vi "GetSwerveEncoders.vi"() -> (16 "Swerve 0 Velocity (ft/s)":dbl, 17 "Swerve 3 Velocity (ft/s)":dbl, 18 "Swerve 1 Velocity (ft/s)":dbl, 19 "Swerve 2 Velocity (ft/s)":dbl, 20 "Swerve 0 Azimuth Position (deg)":dbl, 22 "Swerve 1 Azimuth Position (deg)":dbl, 24 "Swerve 2 Azimuth Position (deg)":dbl, 26 "Swerve 3 Azimuth Position (deg)":dbl)   [LabVIEW 2020]
doc: "Gets the drive distance, azimuth position, and velocity encoder readings from all of the swerve modules. This VI is also useful for characterizing the drive system allowing for estimation of the robot acceleration and plotting of the module velocities. Deteremines the true shifter state based on photo-interrupter sensors on each module. Please see sensors.vi for a reading of the true robot ground speed (as this must be calculated after using the module odometry VIs)."
uses:
  sensordata.vi
  driverdata.vi
  GRNF_CTREMotor.vi
  <vilib>/Rock Robotics/WPI/ThirdParty/Phoenix-LabVIEW/Motor Controller/Get/CTRE_Phoenix_MotorController_GetSelectedSensorData.vi
  <vilib>/Rock Robotics/WPI/ThirdParty/Phoenix-LabVIEW/Motor Controller/Get/CTRE_Phoenix_MotorController_GetLimitSwitchStates.vi
  <vilib>/Rock Robotics/WPI/ThirdParty/Phoenix-LabVIEW/Motor Controller/Get/CTRE_Phoenix_MotorController_GetGeneralStatus.vi
  GlobalDrivebase.vi
panel:
  in  "Shift Time Threshold (ms)":u32=250
  out "Acceleration (ft/s^2)":dbl format="%.1f"
  in  "Reset Acceleration Test":bool
  in  "Plot and Measure":bool
  out "Drive Encoder Velocities (ft/s)":cluster{dbl, dbl, dbl, dbl}(graph)
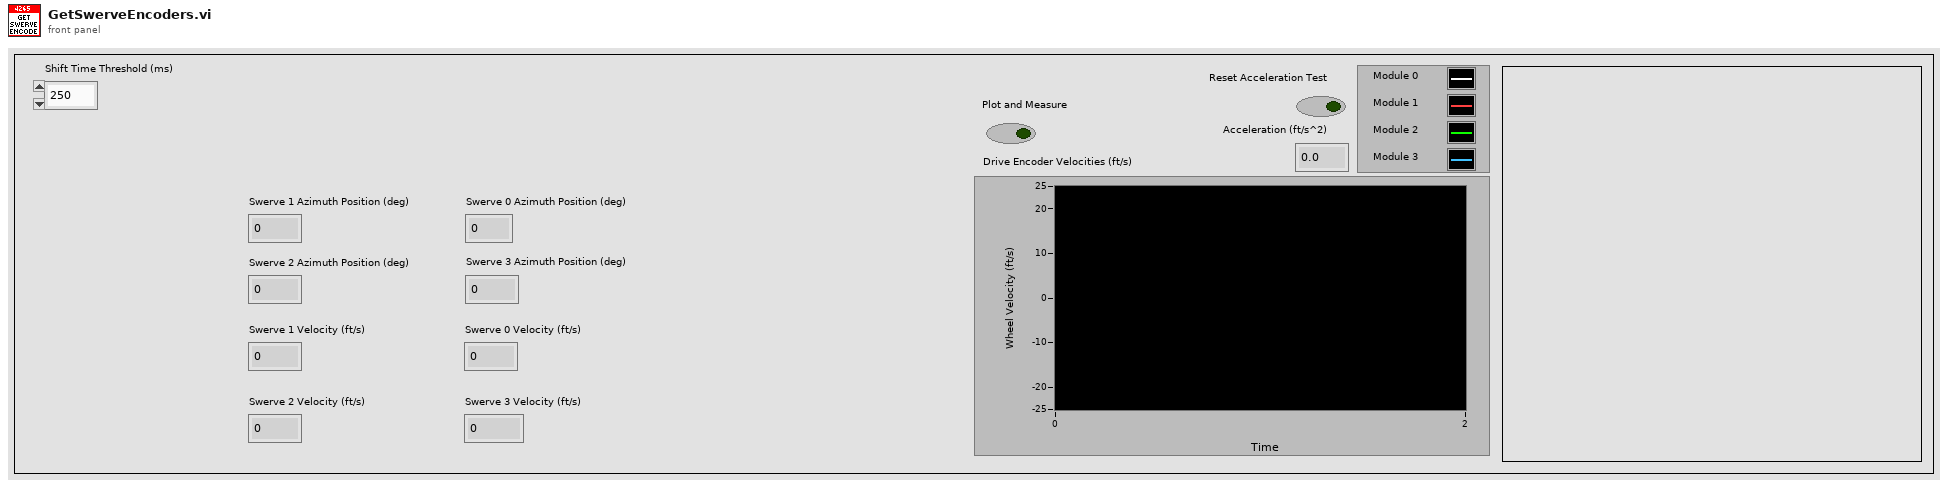
[diagram p1: front panel]
types:
  T1 = typedef "WPI_MotorControlDeviceRef.ctl" = cluster{"DeviceStatus":errorcluster, "Type":T2, "PWM":cluster{"PWM Channel":T3, "DeadBand":T4}, "CAN":cluster{"Device Number":u8, "SetOutput VI Ref":variant, "GetOutput VI Ref":variant, "Enable VI Ref":variant, "Disable VI Ref":variant, "Data":variant}, "Invert":bool, "DIO PWM":cluster{"PWM \"Enable\" Channel":T3, "DIOChannel":T5, "PWM Rate":dbl}}
  T2 = typedef "WPI_MotorControlType.ctl" = enum16{"PWM", "CAN", "DIO PWM"}
  T3 = typedef "FPGA_DIOPWMChannel.ctl" = enum8{"PWM 0", "PWM 1", "PWM 2", "PWM 3", "PWM 4", "PWM 5", "PWM 6", "PWM 7", "PWM 8", "PWM 9", "PWM MXP 0", "PWM MXP 1", "PWM MXP 2", "PWM MXP 3", "PWM MXP 4", "PWM MXP 5", "PWM MXP 6", "PWM MXP 7", "PWM MXP 8", "PWM MXP 9", "Invalid"}
  T4 = typedef "WPI_PWMDeadband.ctl" = cluster{"Name":string, "maxPositivePwm":i32, "minPositivePwm":i32, "centerPwm":i32, "maxNegativePwm":i32, "minNegativePwm":i32, "angularRange":u16}
  T5 = typedef "FPGA_DIOChannel.ctl" = enum8{"DIO 0", "DIO 1", "DIO 2", "DIO 3", "DIO 4", "DIO 5", "DIO 6", "DIO 7", "DIO 8", "DIO 9", "DIO MXP 0", "DIO MXP 1", "DIO MXP 2", "DIO MXP 3", "DIO MXP 4", "DIO MXP 5", "DIO MXP 6", "DIO MXP 7", "DIO MXP 8", "DIO MXP 9", "DIO MXP 10", "DIO MXP 11", "DIO MXP 12", "DIO MXP 13", "DIO MXP 14", "DIO MXP 15", "SPI Port CS1", "SPI Port CS2", "SPI Port CS3", "SPI Port MISO", "SPI Port MOSI", "Invalid"}
  T6 = enum16{"Low Gear", "High Gear", "Transiting", "Unknown", "Force Low Gear"}
  T7 = cluster{"Velocity (ft/s)":dbl, "Velocity (ft/s)":dbl, "Velocity (ft/s)":dbl, "Velocity (ft/s)":dbl}
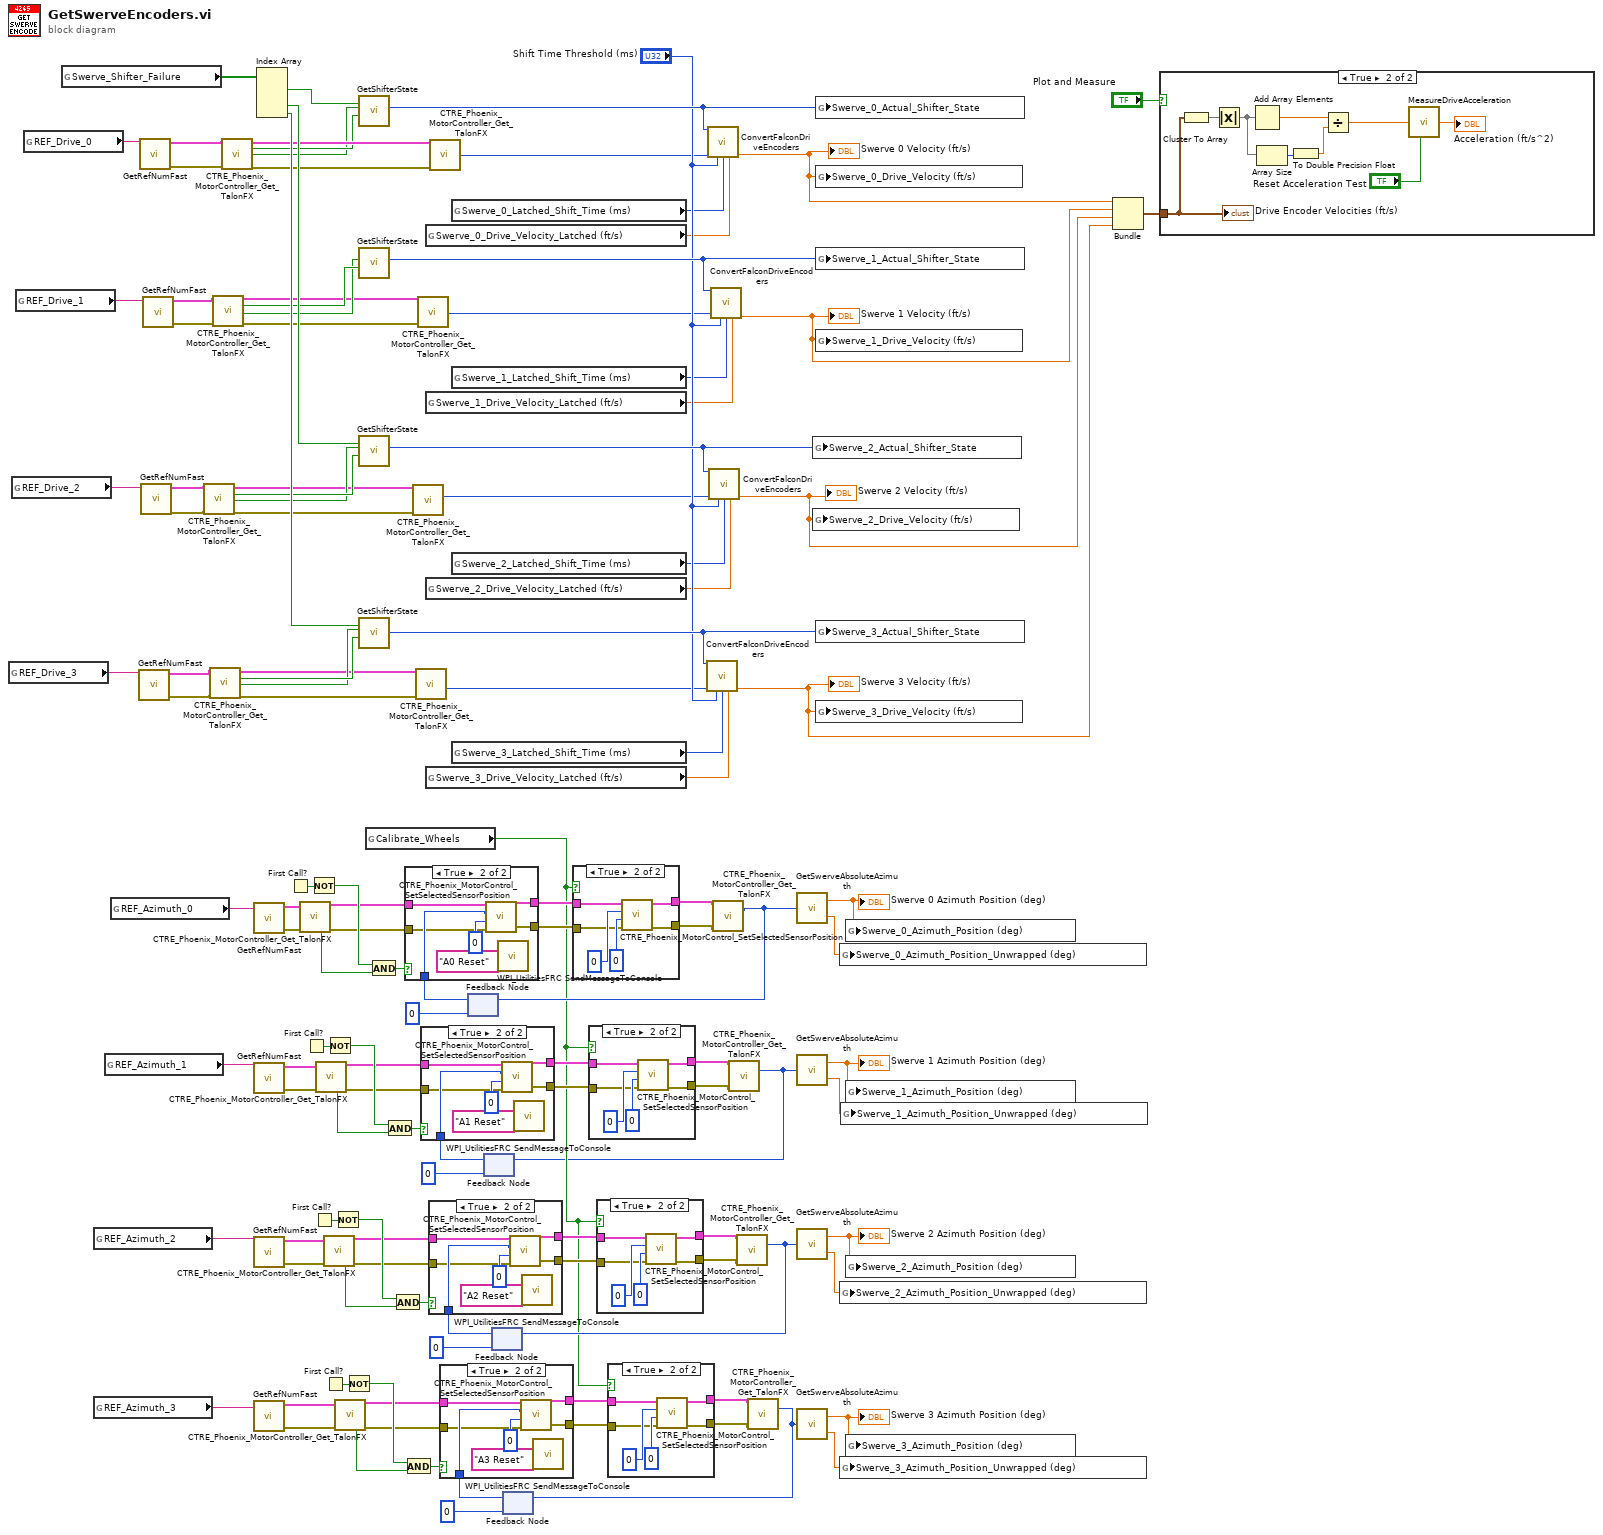
[diagram p0: block diagram]
diagram:
  n1 = global read "GlobalDrivebase.vi" "REF_Drive_3"() -> (w5:string)
  n2 = global read "GlobalDrivebase.vi" "REF_Drive_2"() -> (w6:string)
  n3 = global read "GlobalDrivebase.vi" "REF_Drive_1"() -> (w7:string)
  n4 = global read "GlobalDrivebase.vi" "REF_Drive_0"() -> (w8:string)
  n5 = global read "sensordata.vi" "Swerve_Shifter_Failure"() -> (w122:bool[])
  n6 = global read "GlobalDrivebase.vi" "REF_Azimuth_2"() -> (w2:string)
  n7 = global read "GlobalDrivebase.vi" "REF_Azimuth_3"() -> (w1:string)
  n8 = global read "GlobalDrivebase.vi" "REF_Azimuth_1"() -> (w3:string)
  n9 = global read "GlobalDrivebase.vi" "REF_Azimuth_0"() -> (w4:string)
  n10 = call-poly "GetRefNumFast.vi"("RefNum Name"=w5) -> ("Error"=w16:errorcluster, "Device Reference"=w15:T1)  [unwired: 5 in]
  n11 = call-poly "GetRefNumFast.vi"("RefNum Name"=w8) -> ("Error"=w34:errorcluster, "Device Reference"=w33:T1)  [unwired: 5 in]
  n12 = call-poly "GetRefNumFast.vi"("RefNum Name"=w6) -> ("Error"=w22:errorcluster, "Device Reference"=w21:T1)  [unwired: 5 in]
  n13 = call-poly "GetRefNumFast.vi"("RefNum Name"=w7) -> ("Error"=w31:errorcluster, "Device Reference"=w32:T1)  [unwired: 5 in]
  n14 = call-poly <vilib>:"CTRE_Phoenix_MotorController_Get_TalonFX.vi"("PhoenixMotorControlDevRef"=w21, "error in"=w22) -> ("PhoenixMotorControlDevRef"=w24:T1, "Forward Limit Closed?"=w26:bool, "Reverse Limit Closed?"=w25:bool, "error out"=w23:errorcluster)  [unwired: 10 in]
  n15 = call-poly <vilib>:"CTRE_Phoenix_MotorController_Get_TalonFX.vi"("PhoenixMotorControlDevRef"=w15, "error in"=w16) -> ("PhoenixMotorControlDevRef"=w18:T1, "Forward Limit Closed?"=w20:bool, "Reverse Limit Closed?"=w19:bool, "error out"=w17:errorcluster)  [unwired: 10 in]
  n16 = call-poly <vilib>:"CTRE_Phoenix_MotorController_Get_TalonFX.vi"("PhoenixMotorControlDevRef"=w32, "error in"=w31) -> ("PhoenixMotorControlDevRef"=w28:T1, "Forward Limit Closed?"=w30:bool, "Reverse Limit Closed?"=w29:bool, "error out"=w27:errorcluster)  [unwired: 10 in]
  n17 = call-poly <vilib>:"CTRE_Phoenix_MotorController_Get_TalonFX.vi"("PhoenixMotorControlDevRef"=w33, "error in"=w34) -> ("PhoenixMotorControlDevRef"=w37:T1, "Forward Limit Closed?"=w36:bool, "Reverse Limit Closed?"=w13:bool, "error out"=w35:errorcluster)  [unwired: 10 in]
  n18 = call-poly "GetRefNumFast.vi"("RefNum Name"=w4) -> ("Error"=w93:errorcluster, "Device Reference"=w94:T1)  [unwired: 5 in]
  n19 = call-poly "GetRefNumFast.vi"("RefNum Name"=w3) -> ("Error"=w78:errorcluster, "Device Reference"=w79:T1)  [unwired: 5 in]
  n20 = call-poly "GetRefNumFast.vi"("RefNum Name"=w2) -> ("Error"=w64:errorcluster, "Device Reference"=w65:T1)  [unwired: 5 in]
  n21 = call-poly "GetRefNumFast.vi"("RefNum Name"=w1) -> ("Error"=w49:errorcluster, "Device Reference"=w50:T1)  [unwired: 5 in]
  n22 = Index Array(array=w122) -> (element #1=w121:bool, element #3=w120:bool, element #4=w119:bool)  [unwired: 4 in, 1 out]
  n23 = First Call?() -> (First Call?: T/F=w97:bool)
  n24 = call-poly <vilib>:"CTRE_Phoenix_MotorController_Get_TalonFX.vi"("PhoenixMotorControlDevRef"=w94, "error in"=w93) -> ("PhoenixMotorControlDevRef"=w92:T1, "Has Reset Occurred?"=w90:bool, "error out"=w91:errorcluster)  [unwired: 8 in, 3 out]
  n25 = First Call?() -> (First Call?: T/F=w82:bool)
  n26 = Not(x=w97) -> (.not. x?=w95:bool)
  n27 = First Call?() -> (First Call?: T/F=w68:bool)
  n28 = call-poly <vilib>:"CTRE_Phoenix_MotorController_Get_TalonFX.vi"("PhoenixMotorControlDevRef"=w79, "error in"=w78) -> ("PhoenixMotorControlDevRef"=w77:T1, "Has Reset Occurred?"=w75:bool, "error out"=w76:errorcluster)  [unwired: 8 in, 3 out]
  n29 = First Call?() -> (First Call?: T/F=w53:bool)
  n30 = call-poly <vilib>:"CTRE_Phoenix_MotorController_Get_TalonFX.vi"("PhoenixMotorControlDevRef"=w65, "error in"=w64) -> ("PhoenixMotorControlDevRef"=w63:T1, "Has Reset Occurred?"=w61:bool, "error out"=w62:errorcluster)  [unwired: 8 in, 3 out]
  n31 = Not(x=w82) -> (.not. x?=w80:bool)
  n32 = Not(x=w68) -> (.not. x?=w66:bool)
  n33 = call-poly <vilib>:"CTRE_Phoenix_MotorController_Get_TalonFX.vi"("PhoenixMotorControlDevRef"=w50, "error in"=w49) -> ("PhoenixMotorControlDevRef"=w48:T1, "Has Reset Occurred?"=w46:bool, "error out"=w47:errorcluster)  [unwired: 8 in, 3 out]
  n34 = Not(x=w53) -> (.not. x?=w51:bool)
  n35 = call "GetShifterState.vi"("Sensor Failure"=w121, "Low Gear Sensor"=w36, "High Gear Sensor"=w13) -> ("Actual Shifter State"=w113:T6)  [unwired: 8 in]
  n36 = call "GetShifterState.vi"("Low Gear Sensor"=w30, "High Gear Sensor"=w29) -> ("Actual Shifter State"=w114:T6)  [unwired: 9 in]
  n37 = call "GetShifterState.vi"("Sensor Failure"=w120, "Low Gear Sensor"=w26, "High Gear Sensor"=w25) -> ("Actual Shifter State"=w112:T6)  [unwired: 8 in]
  n38 = call "GetShifterState.vi"("Sensor Failure"=w119, "Low Gear Sensor"=w20, "High Gear Sensor"=w19) -> ("Actual Shifter State"=w111:T6)  [unwired: 8 in]
  n39 = global read "driverdata.vi" "Calibrate_Wheels"() -> (w43:bool)
  n40 = And(x=w95, y=w90) -> (x .and. y?=w98:bool)
  n41 = And(x=w80, y=w75) -> (x .and. y?=w83:bool)
  n42 = And(x=w66, y=w61) -> (x .and. y?=w69:bool)
  n43 = And(x=w51, y=w46) -> (x .and. y?=w54:bool)
  n44 = call-poly <vilib>:"CTRE_Phoenix_MotorController_Get_TalonFX.vi"("PhoenixMotorControlDevRef"=w24, "error in"=w23) -> ("Velocity (Raw Sensor Units per 100 ms)"=w39:i32)  [unwired: 10 in, 3 out]
  n45 = call-poly <vilib>:"CTRE_Phoenix_MotorController_Get_TalonFX.vi"("PhoenixMotorControlDevRef"=w18, "error in"=w17) -> ("Velocity (Raw Sensor Units per 100 ms)"=w38:i32)  [unwired: 10 in, 3 out]
  n46 = call-poly <vilib>:"CTRE_Phoenix_MotorController_Get_TalonFX.vi"("PhoenixMotorControlDevRef"=w28, "error in"=w27) -> ("Velocity (Raw Sensor Units per 100 ms)"=w40:i32)  [unwired: 10 in, 3 out]
  n47 = global read "sensordata.vi" "Swerve_0_Drive_Velocity_Latched (ft/s)"() -> (w108:dbl)
  n48 = global read "sensordata.vi" "Swerve_1_Drive_Velocity_Latched (ft/s)"() -> (w106:dbl)
  n49 = global read "sensordata.vi" "Swerve_2_Drive_Velocity_Latched (ft/s)"() -> (w104:dbl)
  n50 = global read "sensordata.vi" "Swerve_3_Drive_Velocity_Latched (ft/s)"() -> (w102:dbl)
  n51 = call-poly <vilib>:"CTRE_Phoenix_MotorController_Get_TalonFX.vi"("PhoenixMotorControlDevRef"=w37, "error in"=w35) -> ("Velocity (Raw Sensor Units per 100 ms)"=w41:i32)  [unwired: 10 in, 3 out]
  n52 = global read "sensordata.vi" "Swerve_0_Latched_Shift_Time (ms)"() -> (w109:u32)
  n53 = global read "sensordata.vi" "Swerve_1_Latched_Shift_Time (ms)"() -> (w107:u32)
  n54 = global read "sensordata.vi" "Swerve_2_Latched_Shift_Time (ms)"() -> (w105:u32)
  n55 = global read "sensordata.vi" "Swerve_3_Latched_Shift_Time (ms)"() -> (w103:u32)
  n56 = feedback #1(0 ("Position (Raw Sensor Units)")) -> (w101:i32)
  n57 = case shown="True" w98 {
    tunnel: w91 -> [w129 w133]
    tunnel: w92 -> [w130 w136]
    tunnel: [w130 w132] -> w100
    tunnel: [w129 w131] -> w99
    tunnel: w101 -> [_ w135]
    frame False {
    }
    frame True {
      n58 = call <vilib>:"CTRE_Phoenix_MotorControl_SetSelectedSensorPosition.vi"("error in (no error)"=w133, "pidLoopIdx"=u32 0, "New Sensor Position"=w135, "PhoenixMotorControlDevRef"=w136) -> ("error out"=w131:errorcluster, "PhoenixMotorControlDevRef"=w132:T1)  [unwired: 6 in]
      n59 = call <vilib>:"WPI_UtilitiesFRC SendMessageToConsole.vi"("Message"="A0 Reset") -> ()  [unwired: 14 in, 1 out]
    }
  }
  n60 = feedback #2(0 ("Position (Raw Sensor Units)")) -> (w86:i32)
  n61 = case shown="True" w83 {
    tunnel: w76 -> [w138 w142]
    tunnel: w77 -> [w139 w145]
    tunnel: [w139 w141] -> w85
    tunnel: [w138 w140] -> w84
    tunnel: w86 -> [_ w144]
    frame False {
    }
    frame True {
      n62 = call <vilib>:"CTRE_Phoenix_MotorControl_SetSelectedSensorPosition.vi"("error in (no error)"=w142, "pidLoopIdx"=u32 0, "New Sensor Position"=w144, "PhoenixMotorControlDevRef"=w145) -> ("error out"=w140:errorcluster, "PhoenixMotorControlDevRef"=w141:T1)  [unwired: 6 in]
      n63 = call <vilib>:"WPI_UtilitiesFRC SendMessageToConsole.vi"("Message"="A1 Reset") -> ()  [unwired: 14 in, 1 out]
    }
  }
  n64 = feedback #3(0 ("Position (Raw Sensor Units)")) -> (w72:i32)
  n65 = case shown="True" w69 {
    tunnel: w62 -> [w147 w151]
    tunnel: w63 -> [w148 w154]
    tunnel: [w148 w150] -> w71
    tunnel: [w147 w149] -> w70
    tunnel: w72 -> [_ w153]
    frame False {
    }
    frame True {
      n66 = call <vilib>:"CTRE_Phoenix_MotorControl_SetSelectedSensorPosition.vi"("error in (no error)"=w151, "pidLoopIdx"=u32 0, "New Sensor Position"=w153, "PhoenixMotorControlDevRef"=w154) -> ("error out"=w149:errorcluster, "PhoenixMotorControlDevRef"=w150:T1)  [unwired: 6 in]
      n67 = call <vilib>:"WPI_UtilitiesFRC SendMessageToConsole.vi"("Message"="A2 Reset") -> ()  [unwired: 14 in, 1 out]
    }
  }
  n68 = feedback #4(0 ("Position (Raw Sensor Units)")) -> (w57:i32)
  n69 = case shown="True" w54 {
    tunnel: w47 -> [w156 w160]
    tunnel: w48 -> [w157 w163]
    tunnel: [w157 w159] -> w56
    tunnel: [w156 w158] -> w55
    tunnel: w57 -> [_ w162]
    frame False {
    }
    frame True {
      n70 = call <vilib>:"CTRE_Phoenix_MotorControl_SetSelectedSensorPosition.vi"("error in (no error)"=w160, "pidLoopIdx"=u32 0, "New Sensor Position"=w162, "PhoenixMotorControlDevRef"=w163) -> ("error out"=w158:errorcluster, "PhoenixMotorControlDevRef"=w159:T1)  [unwired: 6 in]
      n71 = call <vilib>:"WPI_UtilitiesFRC SendMessageToConsole.vi"("Message"="A3 Reset") -> ()  [unwired: 14 in, 1 out]
    }
  }
  n72 = case shown="True" w43 {
    tunnel: w99 -> [w165 w167]
    tunnel: w100 -> [w166 w170]
    tunnel: [w166 w171] -> w89
    tunnel: [w165 w172] -> w88
    frame False {
    }
    frame True {
      n73 = call <vilib>:"CTRE_Phoenix_MotorControl_SetSelectedSensorPosition.vi"("error in (no error)"=w167, "pidLoopIdx"=u32 0, "New Sensor Position"=0, "PhoenixMotorControlDevRef"=w170) -> ("error out"=w172:errorcluster, "PhoenixMotorControlDevRef"=w171:T1)  [unwired: 6 in]
    }
  }
  n74 = case shown="True" w43 {
    tunnel: w84 -> [w173 w175]
    tunnel: w85 -> [w174 w178]
    tunnel: [w174 w179] -> w74
    tunnel: [w173 w180] -> w73
    frame False {
    }
    frame True {
      n75 = call <vilib>:"CTRE_Phoenix_MotorControl_SetSelectedSensorPosition.vi"("error in (no error)"=w175, "pidLoopIdx"=u32 0, "New Sensor Position"=0, "PhoenixMotorControlDevRef"=w178) -> ("error out"=w180:errorcluster, "PhoenixMotorControlDevRef"=w179:T1)  [unwired: 6 in]
    }
  }
  n76 = case shown="True" w43 {
    tunnel: w70 -> [w181 w183]
    tunnel: w71 -> [w182 w186]
    tunnel: [w182 w187] -> w60
    tunnel: [w181 w188] -> w59
    frame False {
    }
    frame True {
      n77 = call <vilib>:"CTRE_Phoenix_MotorControl_SetSelectedSensorPosition.vi"("error in (no error)"=w183, "pidLoopIdx"=u32 0, "New Sensor Position"=0, "PhoenixMotorControlDevRef"=w186) -> ("error out"=w188:errorcluster, "PhoenixMotorControlDevRef"=w187:T1)  [unwired: 6 in]
    }
  }
  n78 = case shown="True" w43 {
    tunnel: w55 -> [w189 w191]
    tunnel: w56 -> [w190 w194]
    tunnel: [w190 w195] -> w45
    tunnel: [w189 w196] -> w44
    frame False {
    }
    frame True {
      n79 = call <vilib>:"CTRE_Phoenix_MotorControl_SetSelectedSensorPosition.vi"("error in (no error)"=w191, "pidLoopIdx"=u32 0, "New Sensor Position"=0, "PhoenixMotorControlDevRef"=w194) -> ("error out"=w196:errorcluster, "PhoenixMotorControlDevRef"=w195:T1)  [unwired: 6 in]
    }
  }
  n80 = call "ConvertFalconDriveEncoders.vi"("Shifter State"=w111, "Velocity (Raw Sensor Units per 100 ms)"=w38, "Shift Time Threshold (ms)"="Shift Time Threshold (ms)", "Latched Shift Time (ms)"=w103, "Latched Velocity (ft/s)"=w102) -> ("Velocity (ft/s)"=w123:dbl)  [unwired: 10 in]
  "Swerve 3 Velocity (ft/s)" <- w123
  n81 = call "ConvertFalconDriveEncoders.vi"("Shifter State"=w113, "Velocity (Raw Sensor Units per 100 ms)"=w41, "Shift Time Threshold (ms)"="Shift Time Threshold (ms)", "Latched Shift Time (ms)"=w109, "Latched Velocity (ft/s)"=w108) -> ("Velocity (ft/s)"=w127:dbl)  [unwired: 10 in]
  "Swerve 0 Velocity (ft/s)" <- w127
  n82 = call "ConvertFalconDriveEncoders.vi"("Shifter State"=w112, "Velocity (Raw Sensor Units per 100 ms)"=w39, "Shift Time Threshold (ms)"="Shift Time Threshold (ms)", "Latched Shift Time (ms)"=w105, "Latched Velocity (ft/s)"=w104) -> ("Velocity (ft/s)"=w124:dbl)  [unwired: 10 in]
  "Swerve 2 Velocity (ft/s)" <- w124
  n83 = call "ConvertFalconDriveEncoders.vi"("Shifter State"=w114, "Velocity (Raw Sensor Units per 100 ms)"=w40, "Shift Time Threshold (ms)"="Shift Time Threshold (ms)", "Latched Shift Time (ms)"=w107, "Latched Velocity (ft/s)"=w106) -> ("Velocity (ft/s)"=w125:dbl)  [unwired: 10 in]
  "Swerve 1 Velocity (ft/s)" <- w125
  n84 = call-poly <vilib>:"CTRE_Phoenix_MotorController_Get_TalonFX.vi"("PhoenixMotorControlDevRef"=w89, "error in"=w88) -> ("Position (Raw Sensor Units)"=w87:i32)  [unwired: 10 in, 3 out]
  n85 = feedback-in #1(w87) -> ()
  n86 = call-poly <vilib>:"CTRE_Phoenix_MotorController_Get_TalonFX.vi"("PhoenixMotorControlDevRef"=w74, "error in"=w73) -> ("Position (Raw Sensor Units)"=w14:i32)  [unwired: 10 in, 3 out]
  n87 = feedback-in #2(w14) -> ()
  n88 = call-poly <vilib>:"CTRE_Phoenix_MotorController_Get_TalonFX.vi"("PhoenixMotorControlDevRef"=w60, "error in"=w59) -> ("Position (Raw Sensor Units)"=w58:i32)  [unwired: 10 in, 3 out]
  n89 = feedback-in #3(w58) -> ()
  n90 = call-poly <vilib>:"CTRE_Phoenix_MotorController_Get_TalonFX.vi"("PhoenixMotorControlDevRef"=w45, "error in"=w44) -> ("Position (Raw Sensor Units)"=w42:i32)  [unwired: 10 in, 3 out]
  n91 = feedback-in #4(w42) -> ()
  n92 = call "GetSwerveAbsoluteAzimuth.vi"("Relative Position (Raw Sensor Units)"=w87) -> ("Azimuth Position (deg) [-180,+180]"=w115:dbl, "Current Unwrapped Angle (deg) [-Inf,+Inf]"=w12:dbl)
  "Swerve 0 Azimuth Position (deg)" <- w115
  n93 = call "GetSwerveAbsoluteAzimuth.vi"("Relative Position (Raw Sensor Units)"=w14) -> ("Azimuth Position (deg) [-180,+180]"=w116:dbl, "Current Unwrapped Angle (deg) [-Inf,+Inf]"=w11:dbl)
  "Swerve 1 Azimuth Position (deg)" <- w116
  n94 = call "GetSwerveAbsoluteAzimuth.vi"("Relative Position (Raw Sensor Units)"=w58) -> ("Azimuth Position (deg) [-180,+180]"=w117:dbl, "Current Unwrapped Angle (deg) [-Inf,+Inf]"=w10:dbl)
  "Swerve 2 Azimuth Position (deg)" <- w117
  n95 = call "GetSwerveAbsoluteAzimuth.vi"("Relative Position (Raw Sensor Units)"=w42) -> ("Azimuth Position (deg) [-180,+180]"=w118:dbl, "Current Unwrapped Angle (deg) [-Inf,+Inf]"=w9:dbl)
  "Swerve 3 Azimuth Position (deg)" <- w118
  n96 = global write "sensordata.vi" "Swerve_2_Actual_Shifter_State"(w112) -> ()
  n97 = global write "sensordata.vi" "Swerve_2_Drive_Velocity (ft/s)"(w124) -> ()
  n98 = global write "sensordata.vi" "Swerve_0_Actual_Shifter_State"(w113) -> ()
  n99 = global write "sensordata.vi" "Swerve_0_Drive_Velocity (ft/s)"(w127) -> ()
  n100 = global write "sensordata.vi" "Swerve_1_Actual_Shifter_State"(w114) -> ()
  n101 = global write "sensordata.vi" "Swerve_1_Drive_Velocity (ft/s)"(w125) -> ()
  n102 = global write "sensordata.vi" "Swerve_3_Actual_Shifter_State"(w111) -> ()
  n103 = global write "sensordata.vi" "Swerve_3_Drive_Velocity (ft/s)"(w123) -> ()
  n104 = global write "sensordata.vi" "Swerve_0_Azimuth_Position_Unwrapped (deg)"(w12) -> ()
  n105 = global write "sensordata.vi" "Swerve_2_Azimuth_Position_Unwrapped (deg)"(w10) -> ()
  n106 = global write "sensordata.vi" "Swerve_3_Azimuth_Position_Unwrapped (deg)"(w9) -> ()
  n107 = global write "sensordata.vi" "Swerve_1_Azimuth_Position_Unwrapped (deg)"(w11) -> ()
  n108 = global write "sensordata.vi" "Swerve_0_Azimuth_Position (deg)"(w115) -> ()
  n109 = global write "sensordata.vi" "Swerve_1_Azimuth_Position (deg)"(w116) -> ()
  n110 = global write "sensordata.vi" "Swerve_2_Azimuth_Position (deg)"(w117) -> ()
  n111 = global write "sensordata.vi" "Swerve_3_Azimuth_Position (deg)"(w118) -> ()
  n112 = Bundle("Velocity (ft/s)"=w127, "Velocity (ft/s)"=w125, "Velocity (ft/s)"=w124, "Velocity (ft/s)"=w123) -> (w126:T7)  [unwired: 1 in]
  n113 = case shown="True" "Plot and Measure" {
    tunnel: w126 -> [_ w200]
    frame False {
    }
    frame True {
      n114 = Cluster To Array(cluster=w200) -> (array=w202:dbl[])
      n115 = Absolute Value(x=w202) -> (abs(x)=w205:dbl[])
      n116 = Add Array Elements(numeric array=w205) -> (sum=w201:dbl)
      n117 = Array Size(array=w205) -> (size(s)=w203:i32)
      n118 = To Double Precision Float(number=w203) -> (double precision float=w204:dbl)
      n119 = Divide(x=w201, y=w204) -> (x/y=w199:dbl)
      n120 = call "MeasureDriveAcceleration.vi"("Average Drive Velocity (ft/s)"=w199, "Reset"="Reset Acceleration Test") -> ("Acceleration (ft/s^2)"=→"Acceleration (ft/s^2)":dbl)  [unwired: 3 in]
      "Drive Encoder Velocities (ft/s)" <- w200
    }
  }
